vi "TRABS-calc-2017-SD.vi"(1 "II channel seq":T1, 2 "I channel seq":T1) -> (0 "TRABS":dbl[](array[numeric]))   [LabVIEW 2015]
uses:
  controls/data-cluster.ctl
  globalVarSD.vi
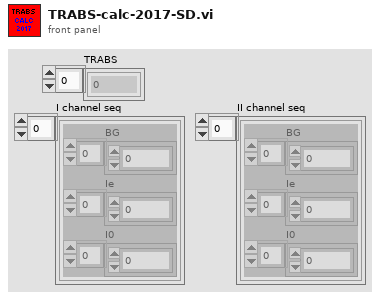
[diagram p1: front panel]
types:
  T1 = typedef "data-cluster.ctl" = cluster{"BG":i32[], "Ie":i32[], "I0":i32[]}[]
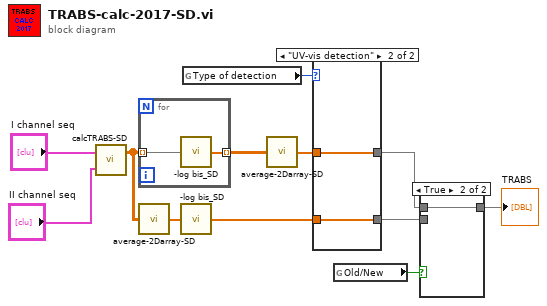
[diagram p0: block diagram]
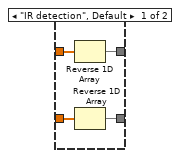
[diagram p3: hidden frame]
diagram:
  n1 = call "calcTRABS-SD.vi"("II channel seq"="II channel seq", "I channel seq"="I channel seq") -> ("TRanS multiple measurements"=w1:dbl[][])  [unwired: 1 out]
  n2 = for {
    tunnel: w1 -> [w14] mode=indexing
    tunnel: [w13] -> w9 mode=indexing
    n3 = call "-log bis_SD.vi"("Transmission"=w14) -> ("-log(x)=log(1/x)"=w13:dbl[])
  }
  n4 = call "average-2Darray-SD.vi"("2D array"=w1) -> ("out array"=w12:dbl[])
  n5 = call "-log bis_SD.vi"("Transmission"=w12) -> ("-log(x)=log(1/x)"=w7:dbl[])
  n6 = global read "globalVarSD.vi" "Type of detection"() -> (w8:enum32{"IR detection", "UV-vis detection"})
  n7 = call "average-2Darray-SD.vi"("2D array"=w9) -> ("out array"=w6:dbl[])
  n8 = case shown="\"UV-vis detection\"" w8 {
    tunnel: w7 -> [w18 w19]
    tunnel: [w17 w19] -> w4
    tunnel: w6 -> [w16 w20]
    tunnel: [w15 w20] -> w3
    frame "IR detection", Default {
      n9 = Reverse 1D Array(array=w16) -> (reversed array=w15:dbl[])
      n10 = Reverse 1D Array(array=w18) -> (reversed array=w17:dbl[])
    }
    frame "UV-vis detection" {
    }
  }
  n11 = global read "globalVarSD.vi" "Old/New"() -> (w5:bool)
  n12 = case shown="True" w5 {
    tunnel: w4 -> [w21 _]
    tunnel: w3 -> [_ w22]
    tunnel: [w21 w22] -> w2
    frame False {
    }
    frame True {
    }
  }
  "TRABS" <- w2
